vi "nWheel to vWheel.vi"(9 "Tire Diameter(m)":fxp<+,16,1>, 11 "nWheel":fxp<+/-,32,16>) -> (2 "vWheel":fxp<+/-,32,18>)   [LabVIEW 2014]
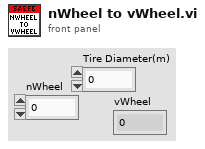
[diagram p1: front panel]
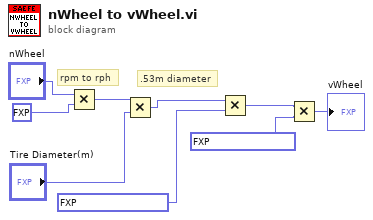
[diagram p0: block diagram]
diagram:
  # ".53m diameter"
  # "rpm to rph"
  n1 = Multiply(x="nWheel", y=fxp<+/-,32,16> 60.0) -> (x*y=w7:fxp<+,32,18>)
  n2 = Multiply(x=w7, y="Tire Diameter(m)") -> (x*y=w5:fxp<+,32,18>)
  n3 = Multiply(x=w5, y=fxp<+/-,32,16> 3.1415863037109375 ("number")) -> (x*y=w2:fxp<+/-,32,19>)
  n4 = Multiply(x=w2, y=fxp<+/-,32,16> 0.001007080078125) -> (x*y=→"vWheel":fxp<+/-,32,18>)
